vi "Connect.vi"(8 "Error In":errorcluster, 10 "Address":string, 11 "Session In":refnum<class "Session.lvclass">) -> (0 "Error Out":errorcluster, 3 "Sesssion Out":refnum<class "Session.lvclass">)   [LabVIEW 2018, in "Toolkit.lvlib" / "Session.lvclass"]
doc: "Connects a sesssion to a remote SSH server. This is typically called immediately after creating the session, and this must be called BEFORE authenticating a user with the remote SSH server."
uses:
  Session.lvclass
  Session.lvclass/Session.ctl
  SSH/SSH.lvclass/SSH.ctl
  Toolkit.lvlib
  SSH/SSH.lvclass
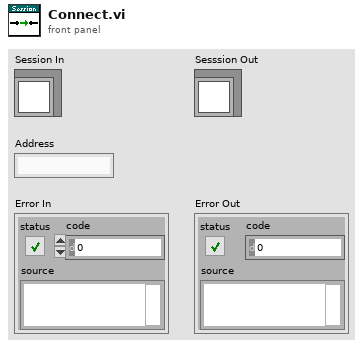
[diagram p1: front panel]
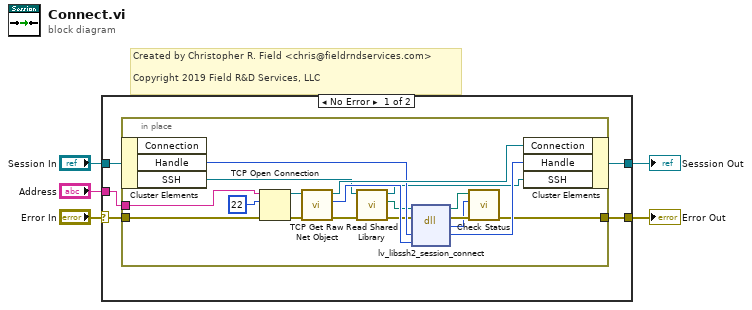
[diagram p0: block diagram]
diagram:
  # "Created by Christopher R. Field <chris@fieldrndservices.com>\n\nCopyright 2019 Field R&D Services, LLC"
  n1 = case shown="No Error" "Error In" {
    selector: "Error In" -> [w8 w30]
    tunnel: "Address" -> [w10 _]
    tunnel: [w9 w30] -> w3
    tunnel: "Session In" -> [w7 w29]
    tunnel: [w6 w29] -> w1
    frame No Error {
      n2 = in-place {
        in-place-border: w10 -> [w27]
        in-place-border: [w16] -> w9
        in-place-border: w8 -> [w26]
        n3 = in-place-cluster #1(w7) -> ("Handle"=w20:u64, "SSH"=w13:refnum<class "SSH.lvclass">)  [unwired: 1 out]
        n4 = TCP Open Connection(address=w27, remote port or service name=u16 22, error in (no error)=w26) -> (connection ID=w24:refnum<k5>, error out=w25:errorcluster)  [unwired: 2 in]
        n5 = call <vilib>:"TCP Get Raw Net Object.vi"("error in (no error)"=w25, "connection ID"=w24) -> ("error out"=w23:errorcluster, "raw net object"=w22:u64, "connection ID out"=w21:refnum<k5>)  [unwired: 7 in]
        n6 = call "Read Shared Library.vi"("Error In"=w23, "SSH In"=w13) -> ("Error Out"=w14:errorcluster, "lv-libssh2 Shared Library"=w11:path, "SSH Out"=w12:refnum<class "SSH.lvclass">)  [unwired: 7 in]
        n7 = dll-call lib="D:/Users/cfield/Code/Field R&D Services/SSH/LV-LIBSSH2/LabVIEW/trunk/src/Toolkit/Support/lv-libssh2.*" fn="lv_libssh2_session_connect"(path in=w11, error in=w14, "session"=w20, "socket"=w22) -> (path out=w17:path, error out=w18:errorcluster, "result"=w15:i32, "session"=w19:u64)  [unwired: 2 in]
        n8 = call "Check Status.vi"("Error In"=w18, "Status"=w15, "lv-libssh2 Shared Library In"=w17) -> ("Error Out"=w16:errorcluster)  [unwired: 7 in, 1 out]
        n9 = in-place-cluster #1("Connection"=w21, "Handle"=w19, "SSH"=w12) -> (w6:refnum<class "Session.lvclass">)
      }
    }
    frame Error {
    }
  }
  "Sesssion Out" <- w1
  "Error Out" <- w3
